vi "Manual.vi"(8 "error in":errorcluster, 10 "Modbus master in":refnum<class "Modbus Master.lvclass">, 11 "Auto Delays":T3={"Agitator Delays"=[], "TF Delays"=[], "Insertion Delays"=[], "Cutting Delays"=[], "PF Delays"=[], "Measur. Delays"=[1000.0], "Reject Delays"=[1000], "BF Delays"=[1000], "P&P Delays"=[1000]}) -> (0 "error out":errorcluster, 1 "OutputCount":u32, 2 "Results":T1, 3 "Auto Times":T2, 5 "Modbus master out":refnum<class "Modbus Master.lvclass">)   [LabVIEW 2021]
uses:
  Controls/Auto Delays.ctl
  Controls/Auto Times.ctl
  <vilib>/Modbus/master/Modbus Master.lvclass
  Controls/Modbus Input.ctl
  Global Variables/RT GV.vi
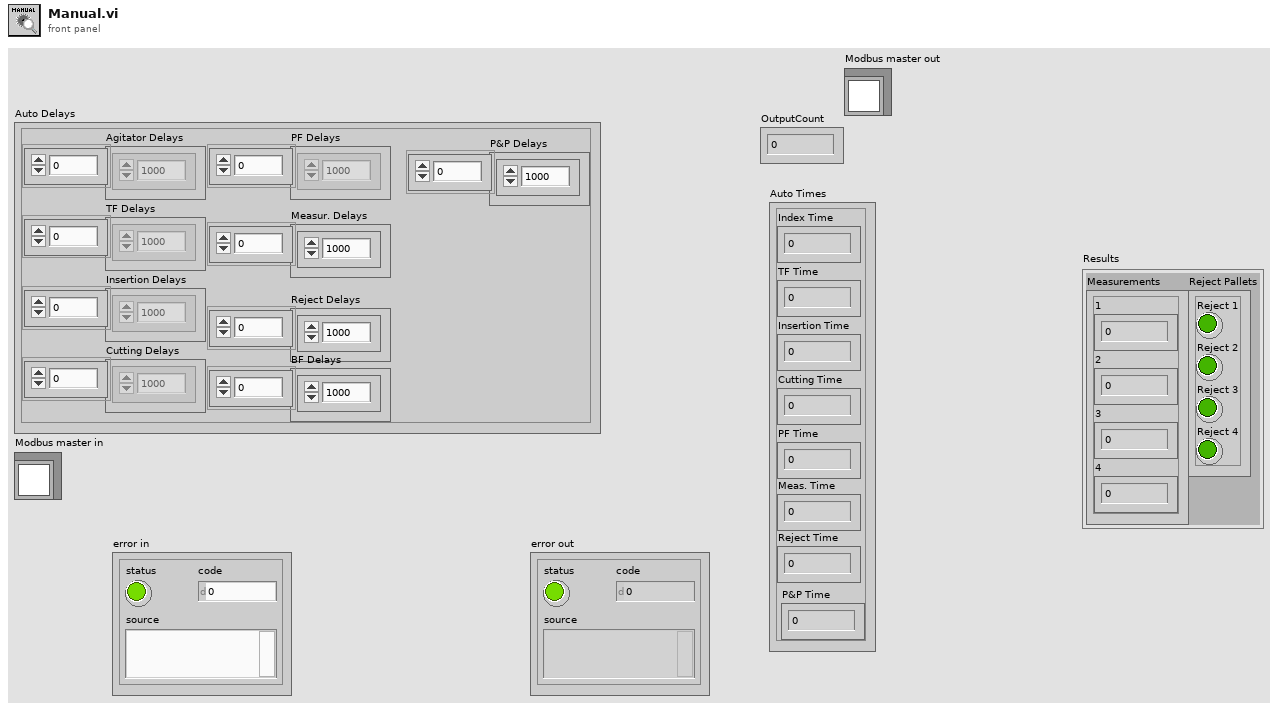
[diagram p1: front panel]
types:
  T1 = cluster{"Measurements":cluster{"1":dbl, "2":dbl, "3":dbl, "4":dbl}, "Reject Pallets":cluster{"Reject 1":bool, "Reject 2":bool, "Reject 3":bool, "Reject 4":bool}}
  T2 = typedef "Auto Times.ctl" = cluster{"Index Time":u32, "TF Time":u32, "Insertion Time":u32, "Cutting Time":u32, "PF Time":u32, "Meas. Time":u32, "Reject Time":u32, "P&P Time":u32}
  T3 = typedef "Auto Delays.ctl" = cluster{"Agitator Delays":u32[], "TF Delays":u32[], "Insertion Delays":u32[], "Cutting Delays":u32[], "PF Delays":u32[], "Measur. Delays":dbl[], "Reject Delays":u32[], "BF Delays":u32[], "P&P Delays":u32[]}
  T4 = typedef "Modbus Input.ctl" = cluster{"Maintenance Mode":bool, "Servo ON":bool, "Start":bool, "Stop":bool, "Reset Fault":bool, "Position Mode":bool, "Velocity Mode":bool, "Index":bool, "Start Index":bool, "Home":bool, "Start":bool, "Maintenance Position":i32, "Maintenance Hardware Torque":u16, "Maintenance Software Torque":u16, "Index Timeout":i16, "Index Position":i32, "Index Hardware Torque Limit":u16, "Index Software Torque Limit":u16, "Homing Timeout":i16, "Prehoming Position":i32, "Prehoming Hardware Torque Limit":u16, "Prehoming Software Torque Limit":u16, "Homing Position":i32, "Homing Hardware Torque Limit":u16, "Homing Software Torque Limit":u16}
  T5 = cluster{"Reject 1":bool, "Reject 2":bool, "Reject 3":bool, "Reject 4":bool}
  T6 = cluster{"Index Time":u32, "TF Time":u32, "Insertion Time":u32, "Cutting Time":u32, "PF Time":u32, "PF Time":u32, "PF Time":u32, "P&P Time":u32}
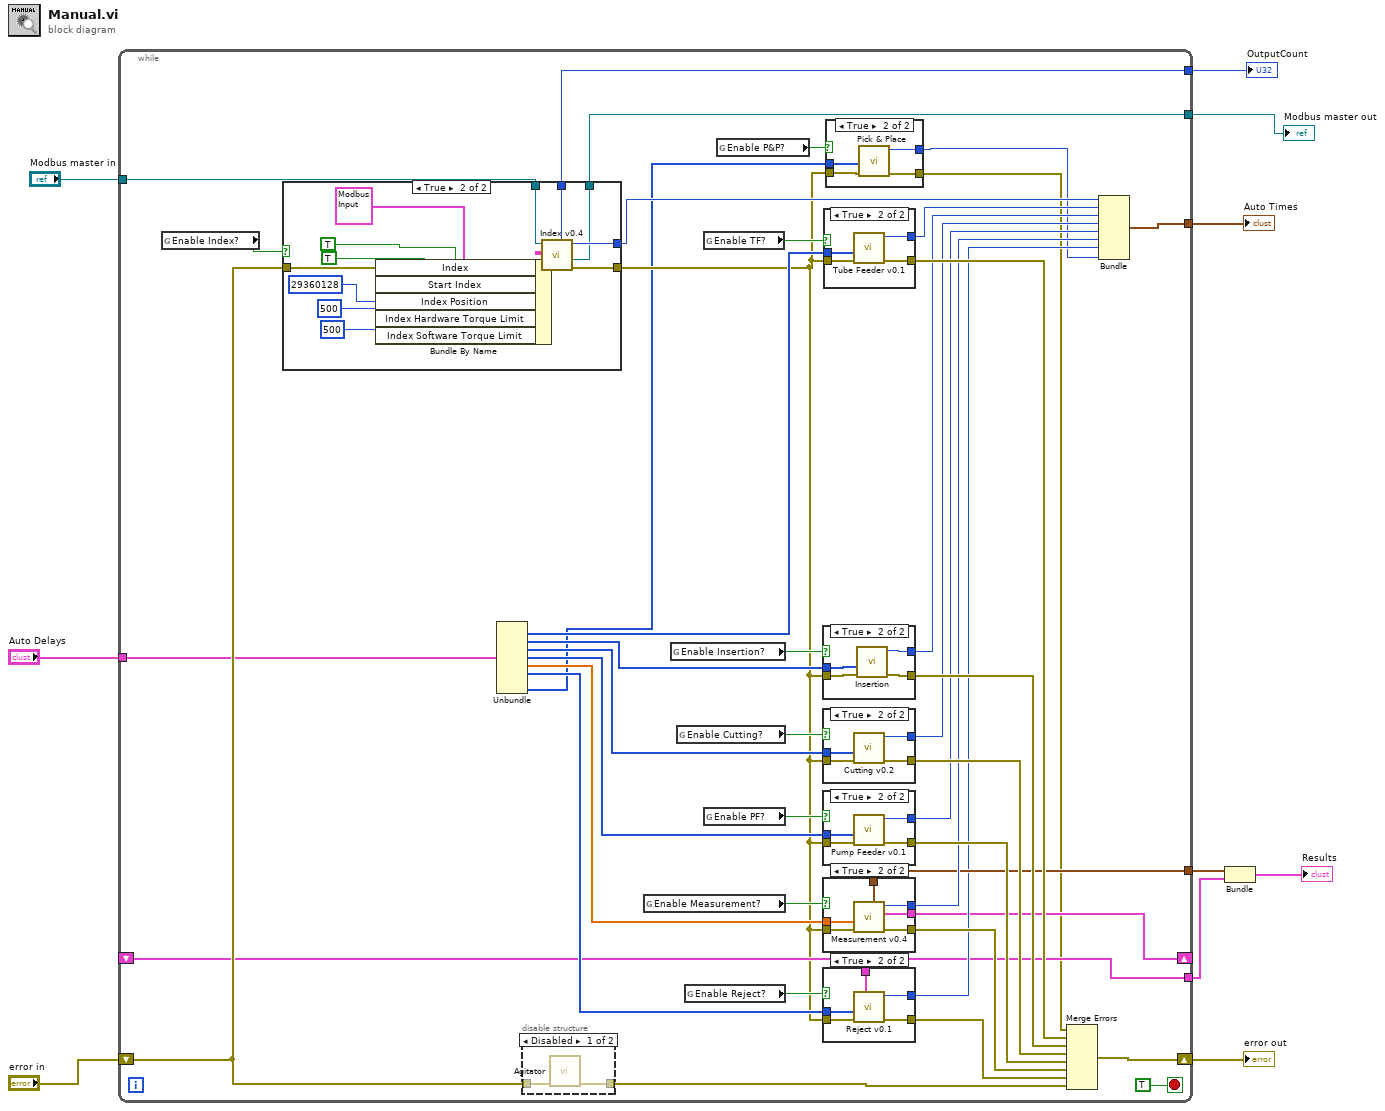
[diagram p0: block diagram]
diagram:
  n1 = while {
    tunnel: "Auto Delays" -> [w45]
    tunnel: [w32] -> w7
    tunnel: [w28] -> w5
    tunnel: [w21] -> w6
    shift-right: [w44] -> w8
    shift-left: "error in" -> [w46]
    shift-right: [w19] -> _
    shift-left: _ -> [w18]
    tunnel: [w18] -> w3
    tunnel: "Modbus master in" -> [w12]
    tunnel: [w11] -> w1
    stop <- TRUE stop-if-true
    n2 = global read "RT GV.vi" "Enable Index?"() -> (w53:bool)
    n3 = case shown="True" w53 {
      tunnel: [w86 w99] -> w17
      tunnel: w46 -> [w86 w98]
      tunnel: [_ w97] -> w37
      tunnel: [_ w96] -> w21
      tunnel: w12 -> [w85 w95]
      tunnel: [w85 w94] -> w11
      frame False {
      }
      frame True {
        n4 = Bundle By Name(cluster=T4 {"Maintenance Mode"=FALSE, "Servo ON"=FALSE, "Start"=FALSE, "Stop"=FALSE, "Reset Fault"=FALSE, "Position Mode"=FALSE, "Velocity Mode"=FALSE, "Index"=FALSE, "Start Index"=FALSE, "Home"=FALSE, "Start"=FALSE, "Maintenance Position"=0, "Maintenance Hardware Torque"=0, "Maintenance Software Torque"=0, "Index Timeout"=0, "Index Position"=0, "Index Hardware Torque Limit"=0, "Index Software Torque Limit"=0, "Homing Timeout"=0, "Prehoming Position"=0, "Prehoming Hardware Torque Limit"=0, "Prehoming Software Torque Limit"=0, "Homing Position"=0, "Homing Hardware Torque Limit"=0, "Homing Software Torque Limit"=0} ("Modbus Input"), "Index"=TRUE, "Start Index"=TRUE, "Index Position"=29360128, "Index Hardware Torque Limit"=u16 500, "Index Software Torque Limit"=u16 500) -> (w92:T4)
        n5 = call "Index v0.4.vi"("error in (no error)"=w98, "Modbus Input"=w92, "Modbus master in"=w95) -> ("error out"=w99:errorcluster, "Modbus master out"=w94:refnum<class "Modbus Master.lvclass">, "Index Time"=w97:u32, "OutputCount"=w96:u32)  [unwired: 4 in, 1 out]
      }
    }
    n6 = Unbundle(w45) -> ("TF Delays"=w49:u32[], "Insertion Delays"=w48:u32[], "Cutting Delays"=w47:u32[], "PF Delays"=w52:u32[], "Measur. Delays"=w30:dbl[], "Reject Delays"=w25:u32[], "P&P Delays"=w13:u32[])  [unwired: 2 out]
    n7 = disable-structure shown="Disabled" {
      disable-tunnel: w46 -> [w60 w61]
      disable-tunnel: [w59 w61] -> w24
      frame Disabled {
        n8 = call "Agitator.vi"("error in (no error)"=w60) -> ("error out"=w59:errorcluster)  [unwired: 9 in, 1 out]
      }
      frame Enabled {
      }
    }
    n9 = global read "RT GV.vi" "Enable Measurement?"() -> (w31:bool)
    n10 = global read "RT GV.vi" "Enable Insertion?"() -> (w42:bool)
    n11 = global read "RT GV.vi" "Enable Cutting?"() -> (w41:bool)
    n12 = global read "RT GV.vi" "Enable Reject?"() -> (w26:bool)
    n13 = global read "RT GV.vi" "Enable TF?"() -> (w43:bool)
    n14 = global read "RT GV.vi" "Enable PF?"() -> (w50:bool)
    n15 = global read "RT GV.vi" "Enable P&P?"() -> (w15:bool)
    n16 = case shown="True" w42 {
      tunnel: w17 -> [w100 w104]
      tunnel: [w100 w103] -> w39
      tunnel: w48 -> [_ w102]
      tunnel: [_ w101] -> w35
      frame False {
      }
      frame True {
        n17 = call "Insertion.vi"("error in (no error)"=w104, "Insertion Delays"=w102) -> ("error out"=w103:errorcluster, "Insertion Time"=w101:u32)  [unwired: 7 in, 1 out]
      }
    }
    n18 = case shown="True" w41 {
      tunnel: w17 -> [w80 w84]
      tunnel: [w80 w83] -> w38
      tunnel: w47 -> [_ w82]
      tunnel: [_ w81] -> w34
      frame False {
      }
      frame True {
        n19 = call "Cutting v0.2.vi"("error in (no error)"=w84, "Cutting Delays"=w82) -> ("error out"=w83:errorcluster, "Cutting Time"=w81:u32)  [unwired: 8 in]
      }
    }
    n20 = case shown="True" w50 {
      tunnel: w17 -> [w75 w79]
      tunnel: [w75 w78] -> w51
      tunnel: w52 -> [_ w77]
      tunnel: [_ w76] -> w33
      frame False {
      }
      frame True {
        n21 = call "Pump Feeder v0.1.vi"("error in (no error)"=w79, "TF Delays"=w77) -> ("error out"=w78:errorcluster, "PF Time"=w76:u32)  [unwired: 8 in]
      }
    }
    n22 = case shown="True" w31 {
      tunnel: w17 -> [w68 w74]
      tunnel: [w68 w73] -> w27
      tunnel: w30 -> [_ w72]
      tunnel: [_ w71] -> w29
      tunnel: [_ w70] -> w28
      tunnel: [_ w69] -> w19
      frame False {
      }
      frame True {
        n23 = call "Measurement v0.4.vi"("error in (no error)"=w74, "TF Delays"=w72) -> ("error out"=w73:errorcluster, "Reject Pallets"=w69:T5, "PF Time"=w71:u32, "Measurements"=w70:cluster{"1":dbl, "2":dbl, "3":dbl, "4":dbl})  [unwired: 5 in, 1 out]
      }
    }
    n24 = case shown="True" w26 {
      tunnel: w17 -> [w62 w67]
      tunnel: [w62 w66] -> w23
      tunnel: w25 -> [_ w65]
      tunnel: [_ w64] -> w22
      tunnel: w18 -> [_ w63]
      frame False {
      }
      frame True {
        n25 = call "Reject v0.1.vi"("Reject Pallets"=w63, "error in (no error)"=w67, "TF Delays"=w65) -> ("error out"=w66:errorcluster, "PF Time"=w64:u32)  [unwired: 7 in]
      }
    }
    n26 = case shown="True" w43 {
      tunnel: w17 -> [w105 w109]
      tunnel: [w105 w108] -> w40
      tunnel: w49 -> [_ w107]
      tunnel: [_ w106] -> w36
      frame False {
      }
      frame True {
        n27 = call "Tube Feeder v0.1.vi"("error in (no error)"=w109, "TF Para"=w107) -> ("error out"=w108:errorcluster, "TF Time"=w106:u32)  [unwired: 8 in]
      }
    }
    n28 = case shown="True" w15 {
      tunnel: w17 -> [w54 w58]
      tunnel: [_ w57] -> w16
      tunnel: [w54 w56] -> w14
      tunnel: w13 -> [_ w55]
      frame False {
      }
      frame True {
        n29 = call "Pick & Place.vi"("error in (no error)"=w58, "P&P Delays"=w55) -> ("error out"=w56:errorcluster, "P&P Time"=w57:u32)  [unwired: 7 in, 1 out]
      }
    }
    n30 = Merge Errors(w14, w40, w39, w38, w51, w27, w23, w24) -> (w44:errorcluster)
    n31 = Bundle("Index Time"=w37, "TF Time"=w36, "Insertion Time"=w35, "Cutting Time"=w34, "PF Time"=w33, "PF Time"=w29, "PF Time"=w22, "P&P Time"=w16) -> (w32:T6)  [unwired: 1 in]
  }
  "error out" <- w8
  "Auto Times" <- w7
  "OutputCount" <- w6
  "Modbus master out" <- w1
  n32 = Bundle("Measurements"=w5, "Reject Pallets"=w3) -> (→"Results":T1)  [unwired: 1 in]
